vi "Write currentBallZone.vi"(8 "error in (no error)":errorcluster, 10 "Enum":T1, 11 "Ally in":refnum<class "Ally.lvclass">) -> (0 "error out":errorcluster, 3 "Ally out":refnum<class "Ally.lvclass">)   [LabVIEW 2023, in "Ally.lvclass"]
uses:
  Ally.lvclass
  Zone_class/zones.ctl
  Ally.lvclass/Ally.ctl
  Zone_class/Zone.lvclass
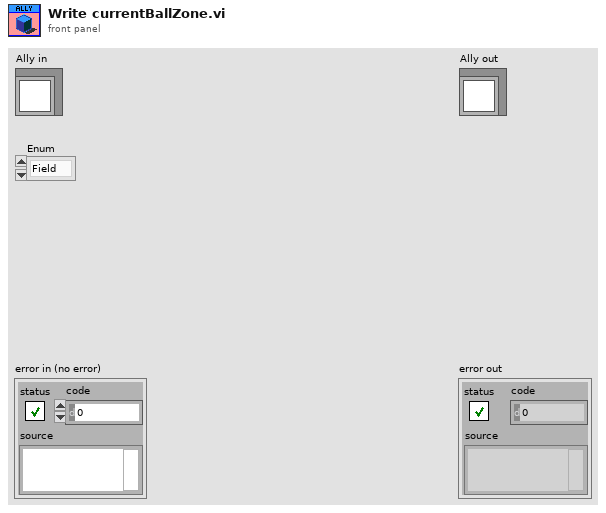
[diagram p1: front panel]
types:
  T1 = typedef "Zone.lvclass/zones.ctl" = enum16{"Field", "LeftSide", "RightSide", "MidField", "LeftForward", "RightForward", "LeftMidField", "RightMidField", "LeftWing", "CenterForward", "RightWing", "Size"}
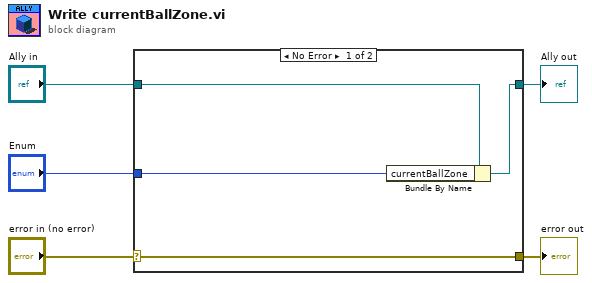
[diagram p0: block diagram]
diagram:
  n1 = case shown="No Error" "error in (no error)" {
    selector: "error in (no error)" -> [w9 w10]
    tunnel: [w9 w10] -> w4
    tunnel: [w7 w11] -> w2
    tunnel: "Ally in" -> [w8 w11]
    tunnel: "Enum" -> [w6 _]
    frame No Error {
      n2 = Bundle By Name(cluster=w8, "currentBallZone"=w6) -> (w7:refnum<class "Ally.lvclass">)
    }
    frame Error {
    }
  }
  "error out" <- w4
  "Ally out" <- w2
